vi "Simulator.vi"() -> ()   [LabVIEW 2017]
uses:
  <vilib>/DAQmx/read.llb/DAQmx Read (Digital 1D Bool NChan 1Samp 1Line).vi
  <vilib>/DAQmx/write.llb/DAQmx Write (Analog Wfm 1Chan NSamp).vi
  <vilib>/DAQmx/create/channels.llb/DAQmx Create Channel (AO-Voltage-Basic).vi
  <vilib>/DAQmx/miscellaneous.llb/DAQmx Fill In Error Info.vi
  <vilib>/DAQmx/create/channels.llb/DAQmx Create Channel (DI-Digital Input).vi
  Variable/Global_simulator.vi
  <vilib>/Utility/file.llb/Write Delimited Spreadsheet (DBL).vi
  <vilib>/Utility/file.llb/Write Delimited Spreadsheet (string).vi
panel:
  out "Y 2":dbl[](array[numeric])
  out "Y":dbl[](array[numeric])
  out "Waveform Chart 2":waveform(dbl)(graph)
  out "Waveform Chart":waveform(dbl)(graph)
  in  "stop":bool
  out "data 3":bool[](array[boolean])
  out "x+y":i16
  out "element":bool
  out "element 2":bool
  out "x+y 2":i16
  in  "File Path Control":path
  in  "delta(ms)":i32
  in  "Off Time(ms)":i32
  in  "No of Rotation":i32
  in  "Dwell Time(ms)":i32
  out "Square":waveform(dbl)(graph)
  in  "Frequency(Hz)":dbl=20.0 caption="Frequency"
  in  "Duty Cycle (%)":dbl=50.0
  # "Signal Generator"
  # "Test Properties"
  # "Signal Properties"
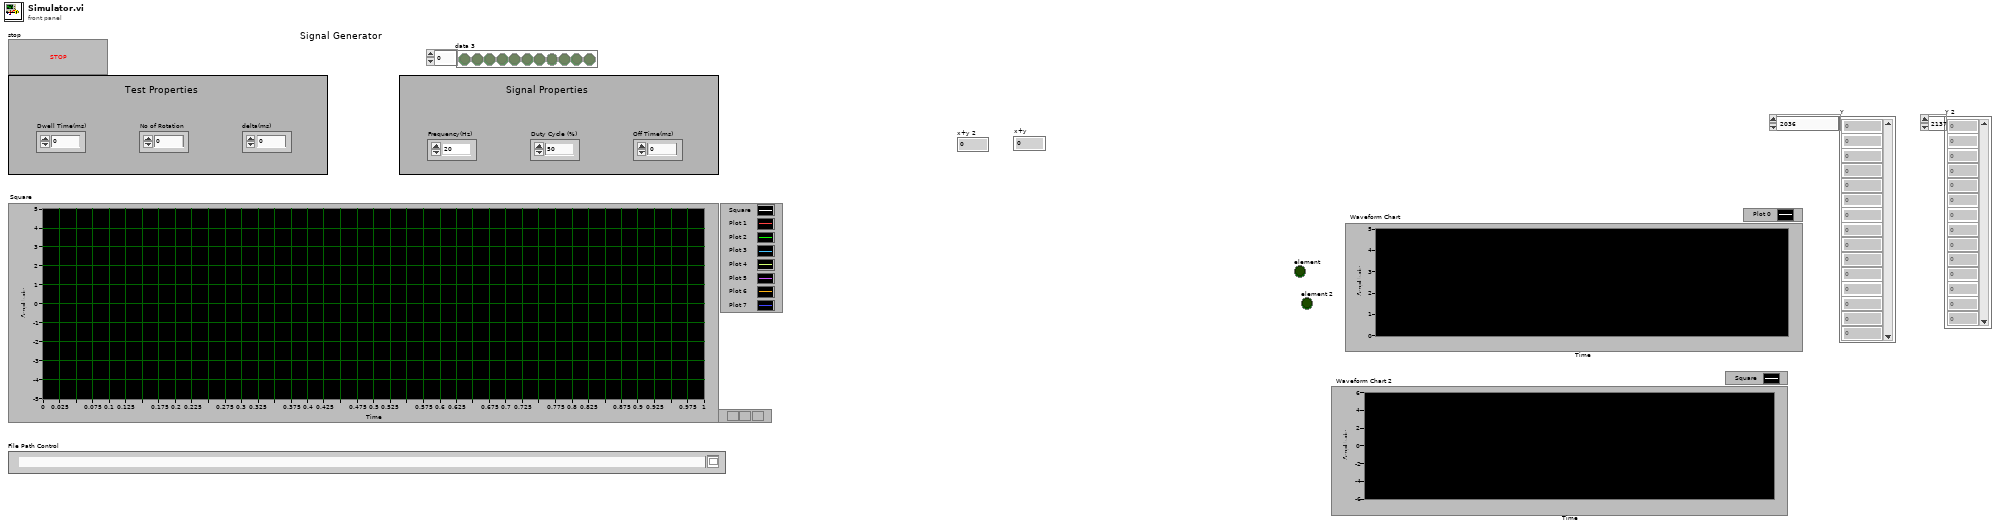
[diagram p1: front panel]
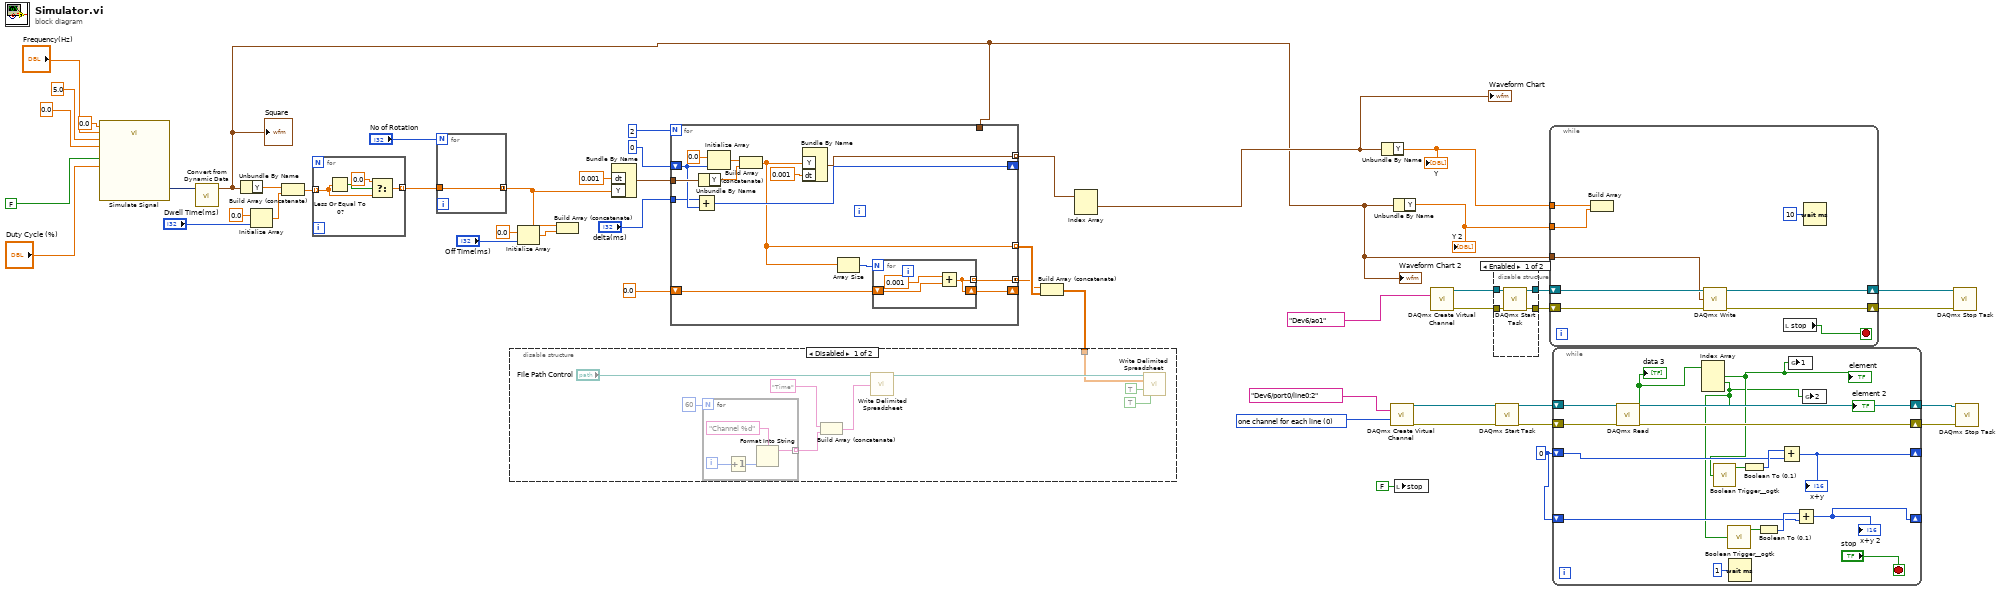
[diagram p0: block diagram]
diagram:
  w8 = 0 items=["one channel for each line", "one channel for all lines"] ("line grouping")
  w7 = i16 0
  n1 = call "Simulate Signal"("Offset"=0.0, "Duty Cycle (%)"="Duty Cycle (%)", "Reset Signal"=FALSE, "Frequency"="Frequency(Hz)", "Amplitude"=5.0, "Phase"=0.0) -> ("Square"=w43:dynamicdata)  [unwired: 8 in, 1 out]
  n2 = call "Convert from Dynamic Data"("Dynamic Data Type"=w43) -> ("Waveform"=w1:waveform(dbl))  [unwired: 3 in]
  "Square" <- w1
  "Waveform Chart 2" <- w1
  n3 = Unbundle By Name(w1) -> ("Y"=w39:dbl[])
  n4 = Initialize Array(0.0 ("element"), "Dwell Time(ms)") -> (w38:dbl[])
  n5 = Build Array (concatenate)(w39, w38) -> (w36:dbl[])
  n6 = for {
    tunnel: w36 -> [w51] mode=indexing
    tunnel: [w50] -> w35 mode=indexing
    n7 = Less Or Equal To 0?(x=w51) -> (x <= 0?=w53:bool)
    n8 = Select(t=0.0, s=w53, f=w51) -> (s? t:f=w50:dbl)
  }
  n9 = for {
    N: "No of Rotation" -> [_]
    tunnel: w35 -> [w54]
    tunnel: [w54] -> w3 mode=concatenating
  }
  n10 = Initialize Array(0.0 ("element"), "Off Time(ms)") -> (w32:dbl[])
  n11 = Build Array (concatenate)(w3, w32) -> ()  [unwired: 1 out]
  n12 = Bundle By Name("dt"=0.001, "Y"=w3) -> (w2:waveform(dbl))  [unwired: 1 in]
  n13 = for {
    N: 2 -> [_]
    tunnel: w2 -> [w68]
    shift-right: [w64] -> _
    shift-left: 0 -> [w66]
    tunnel: "delta(ms)" -> [w65]
    tunnel: [w61] -> w5 mode=indexing
    tunnel: [w58] -> w28 mode=indexing
    tunnel: [w57] -> w27 mode=concatenating
    shift-right: [w55] -> _
    shift-left: 0.0 ("dt") -> [w56]
    tunnel: w1 -> [_]
    n14 = Add(x=w65, y=w66) -> (x+y=w64:i32)
    n15 = Unbundle By Name(w68) -> ("Y"=w63:dbl[])
    n16 = Initialize Array(0.0 ("element"), w66) -> (w62:dbl[])
    n17 = Build Array (concatenate)(w62, w63) -> (w58:dbl[])
    n18 = Bundle By Name("Y"=w58, "dt"=0.001) -> (w61:waveform(dbl))  [unwired: 1 in]
    n19 = Array Size(array=w58) -> (size(s)=w59:i32)
    n20 = for {
      N: w59 -> [_]
      tunnel: [w70] -> w57 mode=indexing
      shift-right: [w70] -> w55
      shift-left: w56 -> [w71]
      n21 = Add(x=0.001 ("dt"), y=w71) -> (x+y=w70:dbl)
    }
  }
  n22 = Build Array (concatenate)(w27, w28) -> (w26:dbl[][])
  n23 = disable-structure shown="Disabled" {
    disable-tunnel: w26 -> [w75 _]
    frame Disabled {
      n24 = for {
        N: 60 -> [_]
        tunnel: [w81] -> w73 mode=indexing
        i -> [w82]
        n25 = Increment(x=w82) -> (x+1=w83:i32)
        n26 = Format Into String(format string="Channel %d", w83) -> (resulting string=w81:string)  [unwired: 2 in, 1 out]
      }
      n27 = Build Array (concatenate)("Time", w73) -> (w72:string[])
      n28 = call-poly <vilib>:"Write Delimited Spreadsheet.vi"("file path (dialog if empty)"="File Path Control", "1D data"=w72) -> ("new file path (Not A Path if cancelled)"=w79:path)  [unwired: 12 in, 1 out]
      n29 = call-poly <vilib>:"Write Delimited Spreadsheet.vi"("file path (dialog if empty)"=w79, "2D data"=w75, "append to file? (new file:F)"=TRUE, "transpose? (no:F)"=TRUE) -> ()  [unwired: 10 in, 2 out]
    }
    frame Enabled {
    }
  }
  n30 = Index Array(array=w5) -> (element #1=w4:waveform(dbl))  [unwired: 2 in, 1 out]
  "Waveform Chart" <- w4
  n31 = Unbundle By Name(w4) -> ("Y"=w10:dbl[])
  "Y" <- w10
  n32 = call-poly <vilib>:"DAQmx Create Virtual Channel.vi"("lines"=tag "Dev6/port0/line0:2", "line grouping"=w8) -> ("task out"=w15:refnum<k21>, "error out"=w13:errorcluster)  [unwired: 12 in]
  n33 = Unbundle By Name(w1) -> ("Y"=w9:dbl[])
  "Y 2" <- w9
  n34 = local write "stop"(FALSE ("stop")) -> ()
  n35 = call-poly <vilib>:"DAQmx Create Virtual Channel.vi"("physical channels"=tag "Dev6/ao1") -> ("task out"=w20:refnum<k21>, "error out"=w19:errorcluster)  [unwired: 13 in]
  n36 = disable-structure shown="Enabled" {
    disable-tunnel: [w88 w89] -> w22
    disable-tunnel: [w87 _] -> w21
    disable-tunnel: w20 -> [w86 w89]
    disable-tunnel: w19 -> [w85 _]
    frame Enabled {
      n37 = call <vilib>:"DAQmx Start Task.vi"("task/channels in"=w86, "error in"=w85) -> ("task out"=w88:refnum<k21>, "error out"=w87:errorcluster)  [unwired: 12 in]
    }
    frame Disabled {
    }
  }
  n38 = call <vilib>:"DAQmx Start Task.vi"("task/channels in"=w15, "error in"=w13) -> ("task out"=w14:refnum<k21>, "error out"=w12:errorcluster)  [unwired: 12 in]
  n39 = while {
    shift-right: [w98] -> w24
    shift-left: w22 -> [w96]
    shift-right: [w97] -> w23
    shift-left: w21 -> [w95]
    tunnel: w10 -> [w92]
    tunnel: w9 -> [w91]
    tunnel: w1 -> [w90]
    stop <- w93 stop-if-true
    n40 = Build Array(w92, w91) -> ()  [unwired: 1 out]
    n41 = call-poly <vilib>:"DAQmx Write.vi"("task/channels in"=w96, "data"=w90, "error in"=w95) -> ("task out"=w98:refnum<k21>, "error out"=w97:errorcluster)  [unwired: 10 in, 1 out]
    n42 = local read "stop"() -> (w93:bool)
    n43 = Wait (ms)(milliseconds to wait=u32 10) -> ()  [unwired: 1 out]
  }
  n44 = while {
    shift-right: [w115] -> w18
    shift-left: w14 -> [w113]
    shift-right: [w114] -> w17
    shift-left: w12 -> [w112]
    shift-right: [w108] -> _
    shift-left: w7 -> [w107]
    shift-right: [w101] -> _
    shift-left: w7 -> [w102]
    stop <- "stop" stop-if-true
    n45 = call-poly <vilib>:"DAQmx Read.vi"("task/channels in"=w113, "error in"=w112) -> ("task out"=w115:refnum<k21>, "data"=w105:bool[], "error out"=w114:errorcluster)  [unwired: 11 in]
    "data 3" <- w105
    n46 = Index Array(array=w105) -> (element #1=w100:bool, element #2=w99:bool)  [unwired: 3 in, 1 out]
    "element" <- w100
    "element 2" <- w99
    n47 = call <userlib>:"Boolean Trigger__ogtk.vi"("Boolean Input"=w100) -> ("Rising Edge"=w106:bool)  [unwired: 1 in, 1 out]
    n48 = call <userlib>:"Boolean Trigger__ogtk.vi"("Boolean Input"=w99) -> ("Rising Edge"=w104:bool)  [unwired: 1 in, 1 out]
    n49 = Wait (ms)(milliseconds to wait=u32 1) -> ()  [unwired: 1 out]
    n50 = Boolean To (0,1)(Boolean=w106) -> (0, 1=w109:i16)
    n51 = Boolean To (0,1)(Boolean=w104) -> (0, 1=w103:i16)
    n52 = Add(x=w109, y=w107) -> (x+y=w108:i16)
    "x+y" <- w108
    n53 = global write "Global_simulator.vi" "1"(w100) -> ()
    n54 = Add(x=w103, y=w102) -> (x+y=w101:i16)
    "x+y 2" <- w101
    n55 = global write "Global_simulator.vi" "2"(w99) -> ()
  }
  n56 = call <vilib>:"DAQmx Stop Task.vi"("task/channels in"=w24, "error in"=w23) -> ()  [unwired: 12 in, 2 out]
  n57 = call <vilib>:"DAQmx Stop Task.vi"("task/channels in"=w18, "error in"=w17) -> ()  [unwired: 12 in, 2 out]
